vi "VFH-get_water_data.vi"(5 "Xi":dbl[](array[numeric]), 7 "Water Temp":dbl=22.0 format="%#_13g") -> (2 "Water Cluster":T1)   [LabVIEW 2020, in "VFH-VNA_File_Handler.lvlib"]
uses:
  VFH-VNA_File_Handler.lvlib
  VFH-file_cluster-r140_water.ctl
panel:
  out "XY Graph 4":cluster{"Frequency":dbl[], "Q [S/m]":dbl[]}(graph)
  out "XY Graph 3":cluster{"Frequency":dbl[], "Permativity'":dbl[]}(graph)
  out "x/y":dbl
  out "x/y 2":dbl
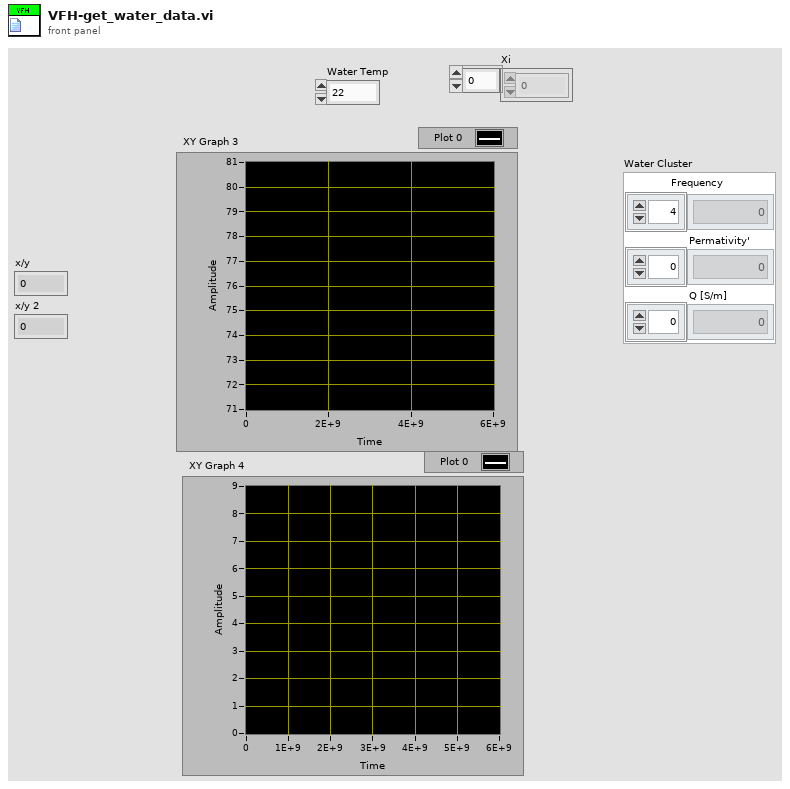
[diagram p1: front panel]
types:
  T1 = typedef "VFH-VNA_File_Handler.lvlib/VFH-file_cluster-r140_water.ctl" = cluster{"Frequency":dbl[], "Permativity'":dbl[], "Q [S/m]":dbl[]}
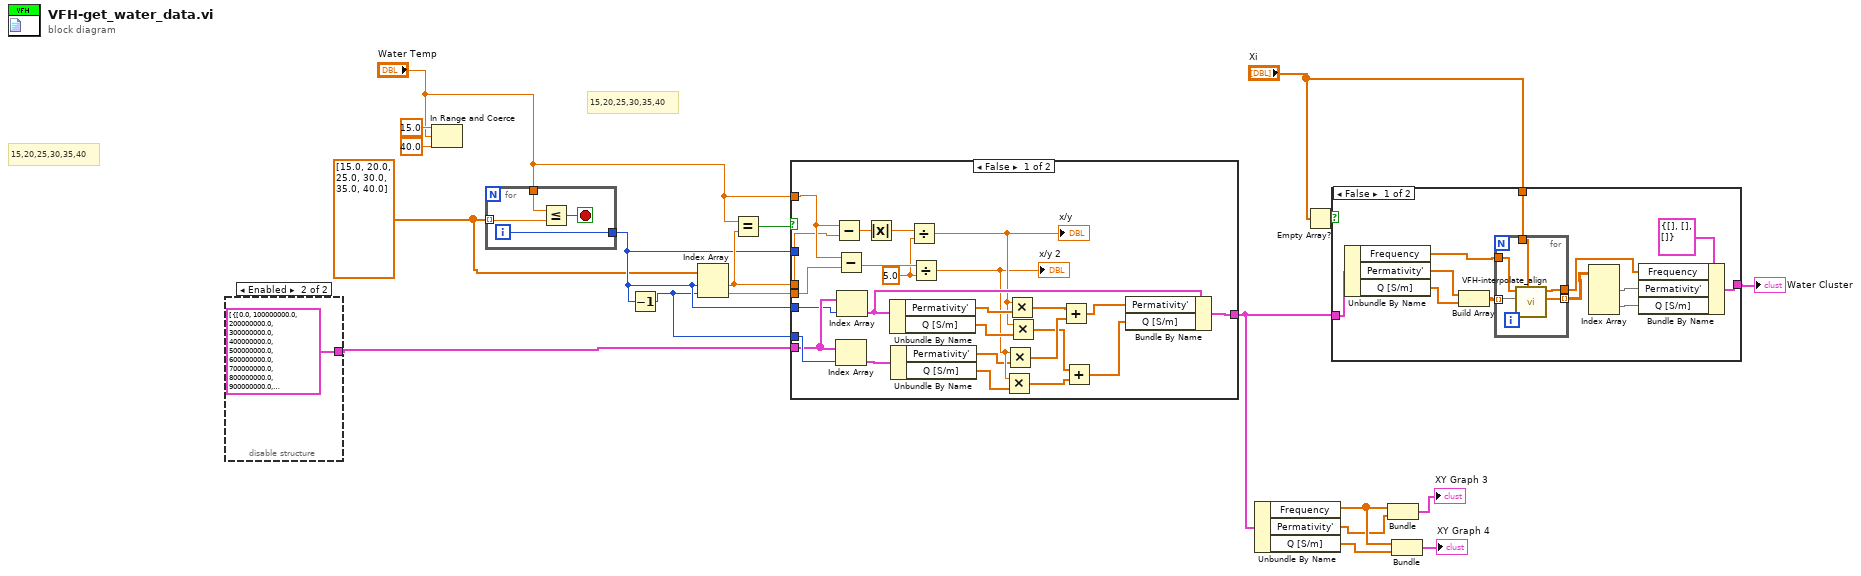
[diagram p0: block diagram]
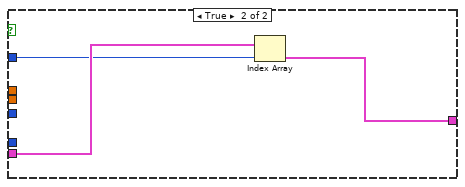
[diagram p3: hidden frame]
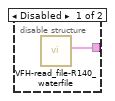
[diagram p4: hidden frame]
diagram:
  w6 = dbl[] [15.0, 20.0, 25.0, 30.0, 35.0, 40.0]
  # "15,20,25,30,35,40"
  # "15,20,25,30,35,40"
  n1 = disable-structure shown="Enabled" {
    disable-tunnel: [w20 T1[] [{"Frequency"=[0.0, 100000000.0, 200000000.0, 300000000.0, 400000000.0, 500000000.0, 600000000.0, 700000000.0, 800000000.0, 900000000.0, 1000000000.0, 1100000000.0, 1200000000.0, 1300000000.0, 1400000000.0, 1500000000.0, 1600000000.0, 1700000000.0, 1800000000.0, 1900000000.0, 2000000000.0, 2100000000.0, 2200000000.0, 2300000000.0, 2400000000.0, 2500000000.0, 2600000000.0, 2700000000.0, 2800000000.0, 2900000000.0, 3000000000.0, 3100000000.0, 3200000000.0, 3300000000.0, 3400000000.0, 3500000000.0, 3600000000.0, 3700000000.0, 3800000000.0, 3900000000.0, 4000000000.0, 4100000000.0, 4200000000.0, 4300000000.0, 4400000000.0, 4500000000.0, 4600000000.0, 4700000000.0, 4800000000.0, 4900000000.0, 5000000000.0, 5100000000.0, 5200000000.0, 5300000000.0, 5400000000.0, 5500000000.0, 5600000000.0, 5700000000.0, 5800000000.0, 5900000000.0], "Permativity'"=[83.92, 83.915, 83.9001, 83.8752, 83.8404, 83.7958, 83.7412, 83.6769, 83.6027, 83.5189, 83.4254, 83.3223, 83.2097, 83.0877, 82.9564, 82.8159, 82.6662, 82.5074, 82.3398, 82.1634, 81.9783, 81.7847, 81.5827, 81.3725, 81.1541, 80.9278, 80.6937, 80.452, 80.2027, 79.9461, 79.6824, 79.4117, 79.1342, 78.8501, 78.5595, 78.2626, 77.9596, 77.6507, 77.3361, 77.0159, 76.6904, 76.3597, 76.024, 75.6834, 75.3383, 74.9887, 74.6349, 74.277, 73.9152, 73.5497, 73.1806, 72.8082, 72.4327, 72.0541, 71.6727, 71.2886, 70.9021, 70.5132, 70.1221, 69.7291], "Q [S/m]"=[0.0, 0.00347541, 0.013899, 0.0312628, 0.0555536, 0.086753, 0.124837, 0.169778, 0.22154, 0.280086, 0.345371, 0.417346, 0.495957, 0.581147, 0.672853, 0.771006, 0.875535, 0.986364, 1.10341, 1.2266, 1.35583, 1.49102, 1.63207, 1.77888, 1.93135, 2.08938, 2.25286, 2.42168, 2.59573, 2.77488, 2.95903, 3.14806, 3.34184, 3.54026, 3.74318, 3.95049, 4.16205, 4.37775, 4.59744, 4.82101, 5.04833, 5.27926, 5.51368, 5.75146, 5.99246, 6.23657, 6.48365, 6.73357, 6.98621, 7.24144, 7.49913, 7.75917, 8.02142, 8.28577, 8.5521, 8.82029, 9.09021, 9.36176, 9.63482, 9.90928]}, {"Frequency"=[0.0, 100000000.0, 200000000.0, 300000000.0, 400000000.0, 500000000.0, 600000000.0, 700000000.0, 800000000.0, 900000000.0, 1000000000.0, 1100000000.0, 1200000000.0, 1300000000.0, 1400000000.0, 1500000000.0, 1600000000.0, 1700000000.0, 1800000000.0, 1900000000.0, 2000000000.0, 2100000000.0, 2200000000.0, 2300000000.0, 2400000000.0, 2500000000.0, 2600000000.0, 2700000000.0, 2800000000.0, 2900000000.0, 3000000000.0, 3100000000.0, 3200000000.0, 3300000000.0, 3400000000.0, 3500000000.0, 3600000000.0, 3700000000.0, 3800000000.0, 3900000000.0, 4000000000.0, 4100000000.0, 4200000000.0, 4300000000.0, 4400000000.0, 4500000000.0, 4600000000.0, 4700000000.0, 4800000000.0, 4900000000.0, 5000000000.0, 5100000000.0, 5200000000.0, 5300000000.0, 5400000000.0, 5500000000.0, 5600000000.0, 5700000000.0, 5800000000.0, 5900000000.0], "Permativity'"=[82.05, 82.0465, 82.0359, 82.0183, 81.9937, 81.9621, 81.9234, 81.8778, 81.8253, 81.7658, 81.6995, 81.6263, 81.5463, 81.4595, 81.366, 81.2659, 81.1591, 81.0458, 80.926, 80.7997, 80.6671, 80.5282, 80.3831, 80.2318, 80.0744, 79.9111, 79.7419, 79.5668, 79.386, 79.1996, 79.0076, 78.8102, 78.6074, 78.3994, 78.1862, 77.968, 77.7448, 77.5167, 77.2839, 77.0465, 76.8045, 76.5582, 76.3075, 76.0526, 75.7936, 75.5307, 75.2638, 74.9933, 74.719, 74.4413, 74.1601, 73.8756, 73.5879, 73.2971, 73.0034, 72.7068, 72.4074, 72.1054, 71.8008, 71.4938], "Q [S/m]"=[0.0, 0.00287872, 0.0115133, 0.0258989, 0.0460275, 0.0718881, 0.103466, 0.140744, 0.183702, 0.232316, 0.286558, 0.3464, 0.411809, 0.482749, 0.55918, 0.641063, 0.728353, 0.821002, 0.918962, 1.02218, 1.1306, 1.24417, 1.36282, 1.4865, 1.61514, 1.74868, 1.88704, 2.03016, 2.17796, 2.33037, 2.48732, 2.64872, 2.8145, 2.98458, 3.15887, 3.3373, 3.51978, 3.70622, 3.89654, 4.09065, 4.28846, 4.48989, 4.69484, 4.90322, 5.11495, 5.32993, 5.54808, 5.76929, 5.99349, 6.22057, 6.45046, 6.68304, 6.91825, 7.15597, 7.39613, 7.63863, 7.88339, 8.1303, 8.3793, 8.63028]}, {"Frequency"=[0.0, 100000000.0, 200000000.0, 300000000.0, 400000000.0, 500000000.0, 600000000.0, 700000000.0, 800000000.0, 900000000.0, 1000000000.0, 1100000000.0, 1200000000.0, 1300000000.0, 1400000000.0, 1500000000.0, 1600000000.0, 1700000000.0, 1800000000.0, 1900000000.0, 2000000000.0, 2100000000.0, 2200000000.0, 2300000000.0, 2400000000.0, 2500000000.0, 2600000000.0, 2700000000.0, 2800000000.0, 2900000000.0, 3000000000.0, 3100000000.0, 3200000000.0, 3300000000.0, 3400000000.0, 3500000000.0, 3600000000.0, 3700000000.0, 3800000000.0, 3900000000.0, 4000000000.0, 4100000000.0, 4200000000.0, 4300000000.0, 4400000000.0, 4500000000.0, 4600000000.0, 4700000000.0, 4800000000.0, 4900000000.0, 5000000000.0, 5100000000.0, 5200000000.0, 5300000000.0, 5400000000.0, 5500000000.0, 5600000000.0, 5700000000.0, 5800000000.0, 5900000000.0], "Permativity'"=[80.21, 80.2074, 80.1997, 80.1868, 80.1687, 80.1455, 80.1172, 80.0838, 80.0452, 80.0015, 79.9528, 79.899, 79.8402, 79.7764, 79.7076, 79.6338, 79.5551, 79.4715, 79.3831, 79.2898, 79.1918, 79.089, 78.9815, 78.8693, 78.7525, 78.6312, 78.5053, 78.3749, 78.2401, 78.1009, 77.9574, 77.8097, 77.6577, 77.5016, 77.3414, 77.1771, 77.0089, 76.8367, 76.6607, 76.4809, 76.2973, 76.1101, 75.9194, 75.725, 75.5273, 75.3261, 75.1216, 74.9138, 74.7028, 74.4888, 74.2716, 74.0515, 73.8285, 73.6027, 73.374, 73.1427, 72.9088, 72.6723, 72.4333, 72.1919], "Q [S/m]"=[0.0, 0.00244105, 0.00976317, 0.0219633, 0.0390365, 0.0609755, 0.0877714, 0.119413, 0.155887, 0.197179, 0.243272, 0.294146, 0.34978, 0.410153, 0.475239, 0.545013, 0.619444, 0.698504, 0.78216, 0.870379, 0.963126, 1.06036, 1.16205, 1.26815, 1.37862, 1.49342, 1.6125, 1.73581, 1.86332, 1.99496, 2.13069, 2.27045, 2.41421, 2.56189, 2.71345, 2.86882, 3.02797, 3.19081, 3.3573, 3.52738, 3.70098, 3.87805, 4.05852, 4.24232, 4.42941, 4.6197, 4.81315, 5.00967, 5.20921, 5.41171, 5.61709, 5.82529, 6.03624, 6.24988, 6.46613, 6.68494, 6.90624, 7.12995, 7.35601, 7.58436]}, {"Frequency"=[0.0, 100000000.0, 200000000.0, 300000000.0, 400000000.0, 500000000.0, 600000000.0, 700000000.0, 800000000.0, 900000000.0, 1000000000.0, 1100000000.0, 1200000000.0, 1300000000.0, 1400000000.0, 1500000000.0, 1600000000.0, 1700000000.0, 1800000000.0, 1900000000.0, 2000000000.0, 2100000000.0, 2200000000.0, 2300000000.0, 2400000000.0, 2500000000.0, 2600000000.0, 2700000000.0, 2800000000.0, 2900000000.0, 3000000000.0, 3100000000.0, 3200000000.0, 3300000000.0, 3400000000.0, 3500000000.0, 3600000000.0, 3700000000.0, 3800000000.0, 3900000000.0, 4000000000.0, 4100000000.0, 4200000000.0, 4300000000.0, 4400000000.0, 4500000000.0, 4600000000.0, 4700000000.0, 4800000000.0, 4900000000.0, 5000000000.0, 5100000000.0, 5200000000.0, 5300000000.0, 5400000000.0, 5500000000.0, 5600000000.0, 5700000000.0, 5800000000.0, 5900000000.0], "Permativity'"=[78.36, 78.358, 78.3521, 78.3422, 78.3284, 78.3107, 78.289, 78.2633, 78.2338, 78.2003, 78.163, 78.1218, 78.0767, 78.0277, 77.9749, 77.9182, 77.8578, 77.7936, 77.7255, 77.6538, 77.5783, 77.4991, 77.4163, 77.3298, 77.2396, 77.1459, 77.0486, 76.9478, 76.8435, 76.7356, 76.6244, 76.5097, 76.3917, 76.2703, 76.1456, 76.0177, 75.8865, 75.7522, 75.6147, 75.4741, 75.3304, 75.1836, 75.0339, 74.8813, 74.7257, 74.5673, 74.4061, 74.2421, 74.0754, 73.906, 73.734, 73.5593, 73.3822, 73.2025, 73.0204, 72.8358, 72.649, 72.4598, 72.2683, 72.0746], "Q [S/m]"=[0.0, 0.00211477, 0.0084584, 0.0190288, 0.0338226, 0.0528351, 0.0760599, 0.10349, 0.135116, 0.170927, 0.210913, 0.255061, 0.303356, 0.355783, 0.412324, 0.472963, 0.53768, 0.606453, 0.679262, 0.756084, 0.836893, 0.921665, 1.01037, 1.10299, 1.19949, 1.29983, 1.404, 1.51195, 1.62366, 1.73908, 1.85819, 1.98095, 2.10732, 2.23727, 2.37075, 2.50772, 2.64815, 2.792, 2.93922, 3.08977, 3.2436, 3.40068, 3.56096, 3.72439, 3.89092, 4.06052, 4.23313, 4.40871, 4.5872, 4.76857, 4.95276, 5.13972, 5.32941, 5.52177, 5.71675, 5.91431, 6.11438, 6.31694, 6.52191, 6.72926]}, {"Frequency"=[0.0, 100000000.0, 200000000.0, 300000000.0, 400000000.0, 500000000.0, 600000000.0, 700000000.0, 800000000.0, 900000000.0, 1000000000.0, 1100000000.0, 1200000000.0, 1300000000.0, 1400000000.0, 1500000000.0, 1600000000.0, 1700000000.0, 1800000000.0, 1900000000.0, 2000000000.0, 2100000000.0, 2200000000.0, 2300000000.0, 2400000000.0, 2500000000.0, 2600000000.0, 2700000000.0, 2800000000.0, 2900000000.0, 3000000000.0, 3100000000.0, 3200000000.0, 3300000000.0, 3400000000.0, 3500000000.0, 3600000000.0, 3700000000.0, 3800000000.0, 3900000000.0, 4000000000.0, 4100000000.0, 4200000000.0, 4300000000.0, 4400000000.0, 4500000000.0, 4600000000.0, 4700000000.0, 4800000000.0, 4900000000.0, 5000000000.0, 5100000000.0, 5200000000.0, 5300000000.0, 5400000000.0, 5500000000.0, 5600000000.0, 5700000000.0, 5800000000.0, 5900000000.0], "Permativity'"=[76.56, 76.5585, 76.554, 76.5466, 76.5361, 76.5227, 76.5063, 76.4869, 76.4646, 76.4393, 76.411, 76.3798, 76.3456, 76.3086, 76.2686, 76.2256, 76.1798, 76.1311, 76.0795, 76.025, 75.9677, 75.9076, 75.8446, 75.7788, 75.7102, 75.6389, 75.5648, 75.4879, 75.4083, 75.3261, 75.2411, 75.1535, 75.0632, 74.9703, 74.8748, 74.7767, 74.6761, 74.5729, 74.4673, 74.3591, 74.2485, 74.1355, 74.02, 73.9022, 73.782, 73.6595, 73.5346, 73.4075, 73.2782, 73.1467, 73.0129, 72.877, 72.739, 72.5988, 72.4566, 72.3124, 72.1661, 72.0178, 71.8676, 71.7155], "Q [S/m]"=[0.0, 0.00181583, 0.00726287, 0.0163397, 0.0290442, 0.045373, 0.0653221, 0.0888864, 0.11606, 0.146836, 0.181208, 0.219165, 0.2607, 0.3058, 0.354457, 0.406656, 0.462386, 0.521632, 0.58438, 0.650614, 0.720319, 0.793477, 0.870069, 0.950079, 1.03349, 1.12027, 1.21041, 1.30388, 1.40066, 1.50074, 1.60408, 1.71065, 1.82045, 1.93343, 2.04957, 2.16885, 2.29124, 2.4167, 2.54522, 2.67675, 2.81128, 2.94876, 3.08918, 3.23249, 3.37866, 3.52767, 3.67948, 3.83405, 3.99135, 4.15135, 4.31402, 4.47931, 4.64719, 4.81763, 4.99059, 5.16604, 5.34393, 5.52423, 5.7069, 5.89192]}, {"Frequency"=[0.0, 100000000.0, 200000000.0, 300000000.0, 400000000.0, 500000000.0, 600000000.0, 700000000.0, 800000000.0, 900000000.0, 1000000000.0, 1100000000.0, 1200000000.0, 1300000000.0, 1400000000.0, 1500000000.0, 1600000000.0, 1700000000.0, 1800000000.0, 1900000000.0, 2000000000.0, 2100000000.0, 2200000000.0, 2300000000.0, 2400000000.0, 2500000000.0, 2600000000.0, 2700000000.0, 2800000000.0, 2900000000.0, 3000000000.0, 3100000000.0, 3200000000.0, 3300000000.0, 3400000000.0, 3500000000.0, 3600000000.0, 3700000000.0, 3800000000.0, 3900000000.0, 4000000000.0, 4100000000.0, 4200000000.0, 4300000000.0, 4400000000.0, 4500000000.0, 4600000000.0, 4700000000.0, 4800000000.0, 4900000000.0, 5000000000.0, 5100000000.0, 5200000000.0, 5300000000.0, 5400000000.0, 5500000000.0, 5600000000.0, 5700000000.0, 5800000000.0, 5900000000.0], "Permativity'"=[74.87, 74.8688, 74.8653, 74.8595, 74.8514, 74.8409, 74.8281, 74.813, 74.7956, 74.7759, 74.7538, 74.7295, 74.7028, 74.6739, 74.6426, 74.6091, 74.5733, 74.5353, 74.495, 74.4524, 74.4076, 74.3605, 74.3112, 74.2597, 74.206, 74.1501, 74.0921, 74.0318, 73.9694, 73.9048, 73.8381, 73.7693, 73.6983, 73.6253, 73.5501, 73.4729, 73.3937, 73.3124, 73.229, 73.1437, 73.0564, 72.9671, 72.8758, 72.7826, 72.6874, 72.5904, 72.4914, 72.3906, 72.2879, 72.1834, 72.077, 71.9689, 71.859, 71.7473, 71.6338, 71.5187, 71.4018, 71.2833, 71.1631, 71.0412], "Q [S/m]"=[0.0, 0.00158519, 0.00634043, 0.0142648, 0.0253567, 0.0396138, 0.0570335, 0.0776121, 0.101346, 0.128229, 0.158257, 0.191425, 0.227724, 0.267148, 0.30969, 0.35534, 0.404089, 0.455929, 0.510849, 0.568837, 0.629883, 0.693975, 0.761099, 0.831244, 0.904394, 0.980537, 1.05966, 1.14174, 1.22677, 1.31472, 1.40559, 1.49936, 1.596, 1.6955, 1.79784, 1.903, 2.01097, 2.12171, 2.23521, 2.35145, 2.47041, 2.59207, 2.71639, 2.84337, 2.97297, 3.10517, 3.23996, 3.3773, 3.51717, 3.65954, 3.80439, 3.9517, 4.10143, 4.25357, 4.40808, 4.56494, 4.72412, 4.88559, 5.04933, 5.21531]}, {"Frequency"=[0.0, 100000000.0, 200000000.0, 300000000.0, 400000000.0, 500000000.0, 600000000.0, 700000000.0, 800000000.0, 900000000.0, 1000000000.0, 1100000000.0, 1200000000.0, 1300000000.0, 1400000000.0, 1500000000.0, 1600000000.0, 1700000000.0, 1800000000.0, 1900000000.0, 2000000000.0, 2100000000.0, 2200000000.0, 2300000000.0, 2400000000.0, 2500000000.0, 2600000000.0, 2700000000.0, 2800000000.0, 2900000000.0, 3000000000.0, 3100000000.0, 3200000000.0, 3300000000.0, 3400000000.0, 3500000000.0, 3600000000.0, 3700000000.0, 3800000000.0, 3900000000.0, 4000000000.0, 4100000000.0, 4200000000.0, 4300000000.0, 4400000000.0, 4500000000.0, 4600000000.0, 4700000000.0, 4800000000.0, 4900000000.0, 5000000000.0, 5100000000.0, 5200000000.0, 5300000000.0, 5400000000.0, 5500000000.0, 5600000000.0, 5700000000.0, 5800000000.0, 5900000000.0], "Permativity'"=[73.18, 73.1791, 73.1763, 73.1717, 73.1652, 73.1568, 73.1467, 73.1346, 73.1208, 73.105, 73.0875, 73.0681, 73.0468, 73.0238, 72.9989, 72.9722, 72.9436, 72.9133, 72.8811, 72.8472, 72.8114, 72.7738, 72.7345, 72.6934, 72.6504, 72.6058, 72.5593, 72.5111, 72.4612, 72.4095, 72.3561, 72.301, 72.2441, 72.1856, 72.1253, 72.0634, 71.9998, 71.9345, 71.8676, 71.799, 71.7287, 71.6569, 71.5834, 71.5083, 71.4317, 71.3534, 71.2736, 71.1922, 71.1093, 71.0248, 70.9388, 70.8513, 70.7623, 70.6718, 70.5799, 70.4865, 70.3916, 70.2953, 70.1976, 70.0985], "Q [S/m]"=[0.0, 0.00140938, 0.00563729, 0.012683, 0.0225455, 0.0352232, 0.0507139, 0.0690152, 0.0901243, 0.114038, 0.140752, 0.170262, 0.202563, 0.237651, 0.27552, 0.316163, 0.359575, 0.405748, 0.454675, 0.506348, 0.560759, 0.6179, 0.677762, 0.740334, 0.805608, 0.873572, 0.944217, 1.01753, 1.0935, 1.17212, 1.25337, 1.33725, 1.42373, 1.5128, 1.60446, 1.69869, 1.79546, 1.89478, 1.99662, 2.10096, 2.2078, 2.31711, 2.42888, 2.5431, 2.65974, 2.77878, 2.90022, 3.02403, 3.15019, 3.27869, 3.40951, 3.54262, 3.67802, 3.81567, 3.95556, 4.09767, 4.24198, 4.38847, 4.53711, 4.68789]}] ("Array 2")] -> w5
    frame Disabled {
      n2 = call "VFH-read_file-R140_waterfile.vi"() -> ("Array"=w20:T1[])  [unwired: 10 in, 1 out]
    }
    frame Enabled {
    }
  }
  n3 = In Range and Coerce(upper limit=15.0, x="Water Temp", lower limit=40.0) -> ()  [unwired: 2 out]
  n4 = for {
    tunnel: w6 -> [w24] mode=indexing
    tunnel: "Water Temp" -> [w25]
    tunnel: [w22] -> w13
    i -> [w22]
    stop <- w23 stop-if-true
    n5 = Less Or Equal?(x=w25, y=w24) -> (x <= y?=w23:bool)
  }
  n6 = Decrement(x=w13) -> (x-1=w12:i32)
  n7 = Index Array(array=w6, index #1=w13, index #2=w12) -> (element #1=w15:dbl, element #2=w14:dbl)
  n8 = Equal?(x="Water Temp", y=w15) -> (x = y?=w17:bool)
  n9 = case shown="False" w17 {
    tunnel: w5 -> [w42 w53]
    tunnel: w13 -> [_ w52]
    tunnel: [w40 w51] -> w2
    tunnel: "Water Temp" -> [w50 _]
    tunnel: w15 -> [w49 _]
    tunnel: w14 -> [w48 _]
    tunnel: w13 -> [w41 _]
    tunnel: w12 -> [w43 _]
    frame False {
      w44 = 5.0 ("y")
      n10 = Subtract(x=w50, y=w49) -> (x-y=w47:dbl)
      n11 = Subtract(x=w50, y=w48) -> (x-y=w45:dbl)
      n12 = Index Array(array=w42, index=w43) -> (element=w38:T1)
      n13 = Index Array(array=w42, index=w41) -> (element=w39:T1)
      n14 = Absolute Value(x=w47) -> (abs(x)=w46:dbl)
      n15 = Unbundle By Name(w39) -> ("Permativity'"=w36:dbl[], "Q [S/m]"=w37:dbl[])
      n16 = Unbundle By Name(w38) -> ("Permativity'"=w33:dbl[], "Q [S/m]"=w32:dbl[])
      n17 = Divide(x=w46, y=w44) -> (x/y=w35:dbl)
      "x/y" <- w35
      n18 = Divide(x=w45, y=w44) -> (x/y=w34:dbl)
      "x/y 2" <- w34
      n19 = Multiply(x=w34, y=w32) -> (x*y=w28:dbl[])
      n20 = Multiply(x=w34, y=w33) -> (x*y=w30:dbl[])
      n21 = Multiply(x=w35, y=w36) -> (x*y=w31:dbl[])
      n22 = Multiply(x=w35, y=w37) -> (x*y=w29:dbl[])
      n23 = Add(x=w31, y=w30) -> (x+y=w26:dbl[])
      n24 = Add(x=w29, y=w28) -> (x+y=w27:dbl[])
      n25 = Bundle By Name(cluster=w39, "Permativity'"=w26, "Q [S/m]"=w27) -> (w40:T1)
    }
    frame True {
      n26 = Index Array(array=w53, index=w52) -> (element=w51:T1)
    }
  }
  n27 = Unbundle By Name(w2) -> ("Frequency"=w10:dbl[], "Permativity'"=w9:dbl[], "Q [S/m]"=w11:dbl[])
  n28 = Empty Array?(array="Xi") -> (empty?=w3:bool)
  n29 = case shown="False" w3 {
    tunnel: "Xi" -> [w62 _]
    tunnel: w2 -> [w61 w71]
    tunnel: [w56 w71] -> w1
    frame False {
      n30 = Unbundle By Name(w61) -> ("Frequency"=w63:dbl[], "Permativity'"=w65:dbl[], "Q [S/m]"=w55:dbl[])
      n31 = Build Array(w65, w55) -> (w64:dbl[][])
      n32 = for {
        tunnel: w64 -> [w66] mode=indexing
        tunnel: w63 -> [w70]
        tunnel: w62 -> [w69]
        tunnel: [w68] -> w58 mode=indexing
        tunnel: [w67] -> w57
        n33 = call "VFH-interpolate_align.vi"("Xi"=w69, "data"=w66, "Frequency"=w70) -> ("data out"=w68:dbl[], "Frequency out"=w67:dbl[])  [unwired: 7 in]
      }
      n34 = Index Array(array=w58) -> (element #1=w59:dbl[], element #2=w60:dbl[])  [unwired: 4 in]
      n35 = Bundle By Name(cluster=T1 {"Frequency"=[], "Permativity'"=[], "Q [S/m]"=[]} ("output cluster"), "Frequency"=w57, "Permativity'"=w59, "Q [S/m]"=w60) -> (w56:T1)
    }
    frame True {
    }
  }
  "Water Cluster" <- w1
  n36 = Bundle("Frequency"=w10, "Permativity'"=w9) -> (→"XY Graph 3":cluster{"Frequency":dbl[], "Permativity'":dbl[]})  [unwired: 1 in]
  n37 = Bundle("Frequency"=w10, "Q [S/m]"=w11) -> (→"XY Graph 4":cluster{"Frequency":dbl[], "Q [S/m]":dbl[]})  [unwired: 1 in]
